vi "checkNum.vi"(8 "error in (no error)":errorcluster, 11 "input string":string) -> (0 "error out":errorcluster, 3 "Is Num":bool)   [LabVIEW 2017]
uses:
  <vilib>/regexp/Match Regular Expression.xnode
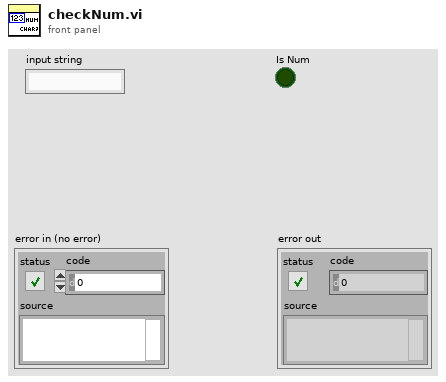
[diagram p1: front panel]
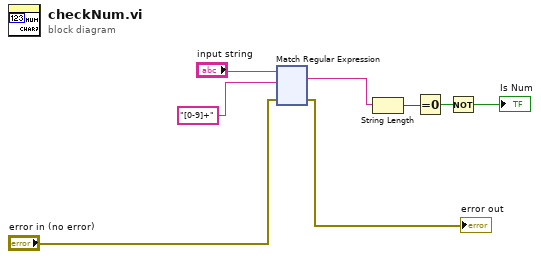
[diagram p0: block diagram]
diagram:
  n1 = xnode "Match Regular Expression"("input string"="input string", "regular expression"="[0-9]+", "error in"="error in (no error)") -> ("whole match"=w4:string, "error out"=→"error out":errorcluster)  [unwired: 3 in, 3 out]
  n2 = String Length(string=w4) -> (length=w3:i32)
  n3 = Equal To 0?(x=w3) -> (x = 0?=w2:bool)
  n4 = Not(x=w2) -> (.not. x?=→"Is Num":bool)
